vi "Created Attributes.vi"(10 "Alias":string, 11 "TEMPLATE Actor in":refnum<class "TEMPLATE Actor.lvclass">) -> (1 "Is Found":bool, 2 "Created Attributes":T1)   [LabVIEW 2020, in "_Template.lvlib" / "Templates.lvlib" / "TEMPLATE Actor.lvlib" / "TEMPLATE Actor.lvclass"]
uses:
  TEMPLATE Actor.lvclass
  jettl/jettl/Actor/Actor/Actor.lvclass
  jettl/jettl/Msg/Msg.lvclass
  jettl/jettl/Actor/Implemented Msgs.ctl
  jettl/jettl/Actor/Actor.lvlib
  jettl/jettl/Actor/Attributes.ctl
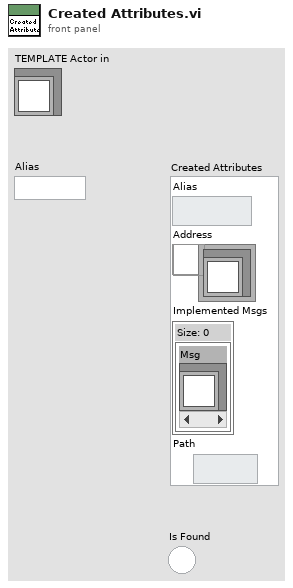
[diagram p1: front panel]
types:
  T1 = typedef "jettl.lvlib/Actor.lvlib/Attributes.ctl" = cluster{"Alias":string, "Address":refnum<user-event>, "Implemented Msgs":T2, "Path":path}
  T2 = typedef "jettl.lvlib/Actor.lvlib/Implemented Msgs.ctl" = set{refnum<class "Msg.lvclass">}
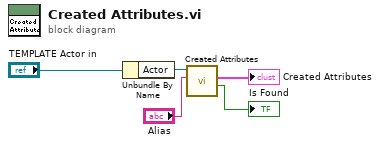
[diagram p0: block diagram]
diagram:
  n1 = Unbundle By Name("TEMPLATE Actor in") -> ("Actor"=w4:refnum<class "Actor.lvclass">)
  n2 = call-dynamic "Created Attributes.vi"("Alias"="Alias", "Actor in"=w4) -> ("Is Found"=→"Is Found":bool, "Created Attributes"=→"Created Attributes":T1)  [unwired: 8 in]
